vi "SDG60ConfNoise.vi"(5 "BandWidth (80 MHz)":dbl=80000000.0 format="%#.3g", 6 "Standard Deviation (0.008 V)":dbl=0.008 format="%#.15g", 7 "Enable BandSet (T:Enable)":bool=TRUE, 8 "error in (no error)":errorcluster, 9 "Mean (0.00 V)":dbl min=-9.996 max=9.996 format="%#.15g", 10 "Channel (1:Channel 1)":i32(ring)=1 items=["Channel 1"=1, "Channel 2"=2], 11 "VISA resource name":refnum<visa-resource-name>="USB0::0xF4EC::0x1101::SDG6XEBC5R0119::INSTR") -> (0 "error out":errorcluster, 3 "VISA resource name out":refnum<visa-resource-name>)   [LabVIEW 2018]
doc: "Configures Noise waveform and parameters."
panel:
  # "Will produce white Gaussian noise"
  # "Range: 20mV-1.19654V\n0.1mV precision"
  # "+-9.98569V"
  # "Bandstate enables you to set the noise \nbandwidth when enabled\nWhen disabled, automatically sets bandwidth"
  # "Min 1mHz\nMax 200 MHz\n10 digits precision"
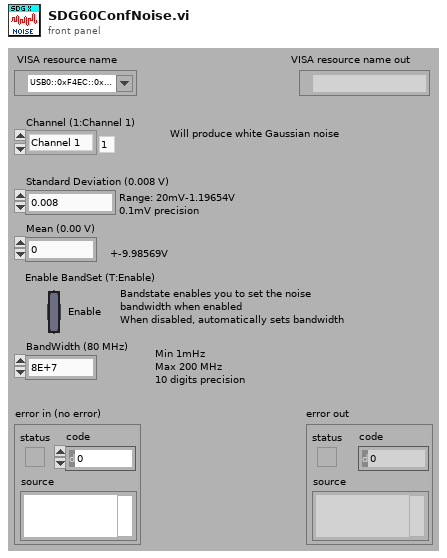
[diagram p1: front panel]
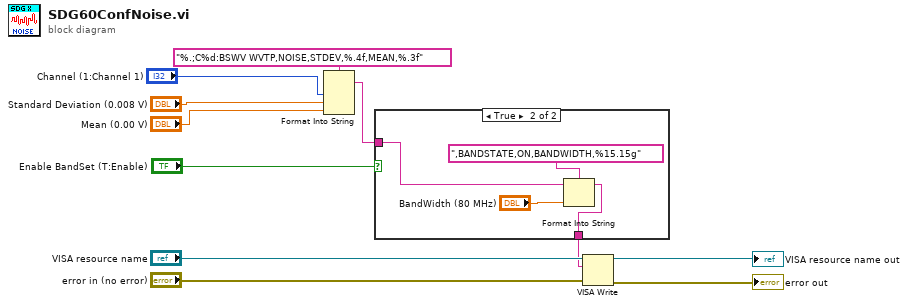
[diagram p0: block diagram]
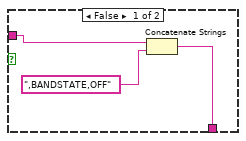
[diagram p2: hidden frame]
diagram:
  n1 = Format Into String(format string="%.;C%d:BSWV WVTP,NOISE,STDEV,%.4f,MEAN,%.3f", "Channel (1:Channel 1)", "Standard Deviation (0.008 V)", "Mean (0.00 V)") -> (resulting string=w5:string)  [unwired: 2 in, 1 out]
  n2 = case shown="True" "Enable BandSet (T:Enable)" {
    tunnel: w5 -> [w14 w16]
    tunnel: [w12 w15] -> w4
    frame False {
      n3 = Concatenate Strings(w14, ",BANDSTATE,OFF" ("格式字符串")) -> (w12:string)
    }
    frame True {
      n4 = Format Into String(format string=",BANDSTATE,ON,BANDWIDTH,%15.15g" ("格式字符串"), initial string=w16, "BandWidth (80 MHz)") -> (resulting string=w15:string)  [unwired: 1 in, 1 out]
    }
  }
  n5 = VISA Write(VISA resource name="VISA resource name", write buffer=w4, error in (no error)="error in (no error)") -> (VISA resource name out=→"VISA resource name out":refnum<visa-resource-name>, error out=→"error out":errorcluster)  [unwired: 1 out]
